vi "题目7.vi"() -> ()   [LabVIEW 2017]
panel:
  out "所用时间（ms）":dbl
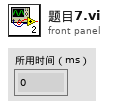
[diagram p1: front panel]
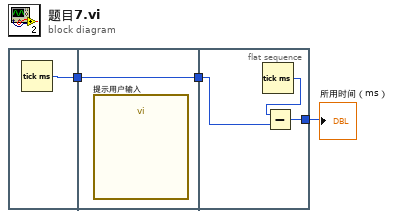
[diagram p0: block diagram]
diagram:
  n1 = flat-sequence {
    tunnel: [w4] -> w3
    tunnel: w3 -> [w5]
    tunnel: [w5] -> w2
    tunnel: w2 -> [w7]
    tunnel: [w6] -> w1
    frame #0 {
      n2 = Tick Count (ms)() -> (millisecond timer value=w4:u32)
    }
    frame #1 {
      n3 = call "提示用户输入"() -> ()  [unwired: 17 in, 3 out]
    }
    frame #2 {
      n4 = Tick Count (ms)() -> (millisecond timer value=w8:u32)
      n5 = Subtract(x=w8, y=w7) -> (x-y=w6:u32)
    }
  }
  "所用时间（ms）" <- w1
